vi "Update Stats.vi"(8 "error in (no error)":errorcluster, 9 "Number Read":i32, 10 "Number Filtered":u32, 11 "L2Enet_RW_CORE in":refnum<class "L2ENET_RW_CORE.lvclass">) -> (0 "error out":errorcluster, 3 "L2Enet_RW_CORE out":refnum<class "L2ENET_RW_CORE.lvclass">)   [LabVIEW 2021, in "L2ENET_RW_CORE.lvclass"]
uses:
  L2ENET_RW_CORE.lvclass
  L2ENET_RW_CORE.lvclass/L2ENET_RW_CORE.ctl
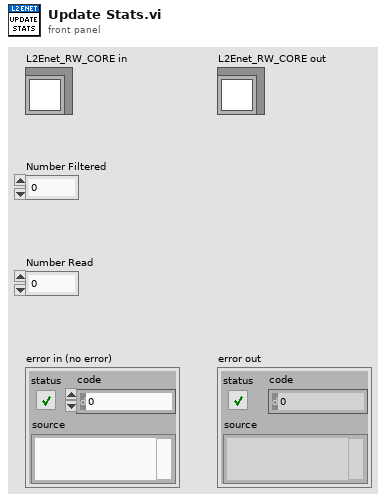
[diagram p1: front panel]
types:
  T1 = typedef "L2ENET_RW_CORE.lvclass/Statistics.ctl" = cluster{"Total Frames RW":u32, "Frames Filtered ":u32}
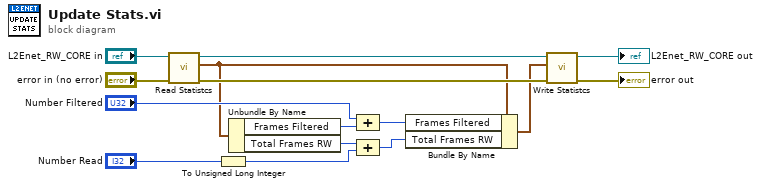
[diagram p0: block diagram]
diagram:
  n1 = call "Read Statistcs.vi"("error in (no error)"="error in (no error)", "CAN_RW_CORE in"="L2Enet_RW_CORE in") -> ("error out"=w12:errorcluster, "Statistcs"=w7:T1, "CAN_RW_CORE out"=w8:refnum<class "L2ENET_RW_CORE.lvclass">)  [unwired: 7 in]
  n2 = To Unsigned Long Integer(number="Number Read") -> (unsigned 32bit integer=w4:u32)
  n3 = Unbundle By Name(w7) -> ("Frames Filtered"=w2:u32, "Total Frames RW"=w6:u32)
  n4 = Compound Arithmetic op=ADD("Number Filtered", w2) -> (w1:u32)
  n5 = Compound Arithmetic op=ADD(w6, w4) -> (w5:u32)
  n6 = Bundle By Name(cluster=w7, "Frames Filtered"=w1, "Total Frames RW"=w5) -> (w3:T1)
  n7 = call "Write Statistcs.vi"("error in (no error)"=w12, "Statistcs"=w3, "CAN_RW_CORE in"=w8) -> ("error out"=→"error out":errorcluster, "CAN_RW_CORE out"=→"L2Enet_RW_CORE out":refnum<class "L2ENET_RW_CORE.lvclass">)  [unwired: 7 in]
